vi "Write Configuration to initialize ACS.vi"(8 "error in (no error)":errorcluster, 10 "Configuration to initialize ACS":T1={"Image path"=path "C:/images/today", "Channel"=1, "S4ACS mode"=0, "Log file path"=path "C:/sparc4/log/s4acs1", "log level"=0} {"log level" items=["DEBBUG", "INFO", "WARNING", "ERROR", "CRITICAL"]; "S4ACS mode" items=["simulated", "real"]; "Channel" min=1 max=4}, 11 "Channel in":refnum<class "Channel.lvclass">) -> (0 "error out":errorcluster, 3 "Channel out":refnum<class "Channel.lvclass">)   [LabVIEW 2018, in "Channel.lvclass"]
uses:
  Channel.lvclass
  Channel.lvclass/Channel.ctl
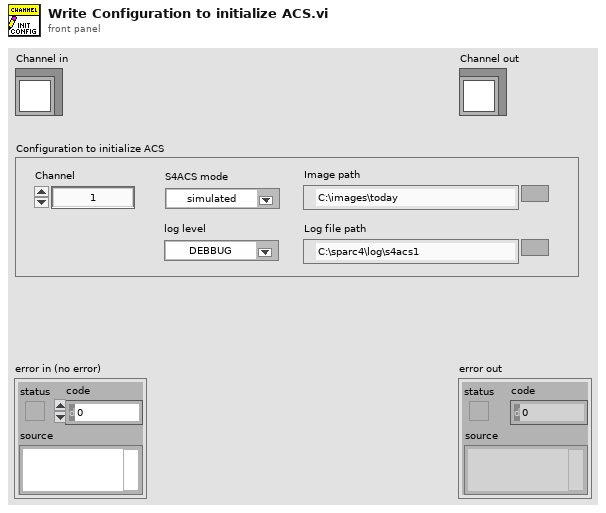
[diagram p1: front panel]
types:
  T1 = cluster{"Image path":path, "Channel":u8, "S4ACS mode":u16, "Log file path":path, "log level":u16}
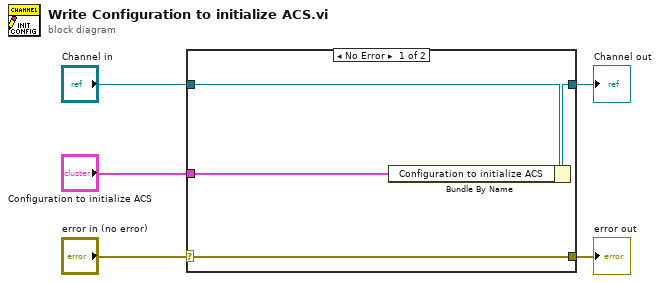
[diagram p0: block diagram]
diagram:
  n1 = case shown="No Error" "error in (no error)" {
    selector: "error in (no error)" -> [w9 w10]
    tunnel: [w9 w10] -> w4
    tunnel: [w7 w11] -> w2
    tunnel: "Channel in" -> [w8 w11]
    tunnel: "Configuration to initialize ACS" -> [w6 _]
    frame No Error {
      n2 = Bundle By Name(cluster=w8, "Configuration to initialize ACS"=w6) -> (w7:refnum<class "Channel.lvclass">)
    }
    frame Error {
    }
  }
  "error out" <- w4
  "Channel out" <- w2
